vi "warmup.vi"(0 "VISA resource name":refnum<visa-resource-name>, 1 "SMU1 Terminal":string(combo)="Source", 5 "error in (no error)":errorcluster, 12 "Sweep 0":T1={"DorG_0"="", "Vvar_0_start"=0.0, "Vvar_0_step"=0.0, "Vvar_0_Stop"=0.0, "Vvar_1_start "=0.0, "Drain Current Compliance"=1e-06, "Gate Current Compliance 0"=1e-06, "Vvar_0_holdtime"=0.0, "Vvar-0_delaytime"=0.0, "IntPts_0"=100.0, "Set Swe_0_Mode"="", "Sweep Spacing_0"=""}) -> (14 "VISA resource name out":refnum<visa-resource-name>, 15 "Recorded_data":dbl[][](array[numeric]), 19 "error out":errorcluster)   [LabVIEW 2021]
panel:
  out "V Slave":string
  out "V Lead":string
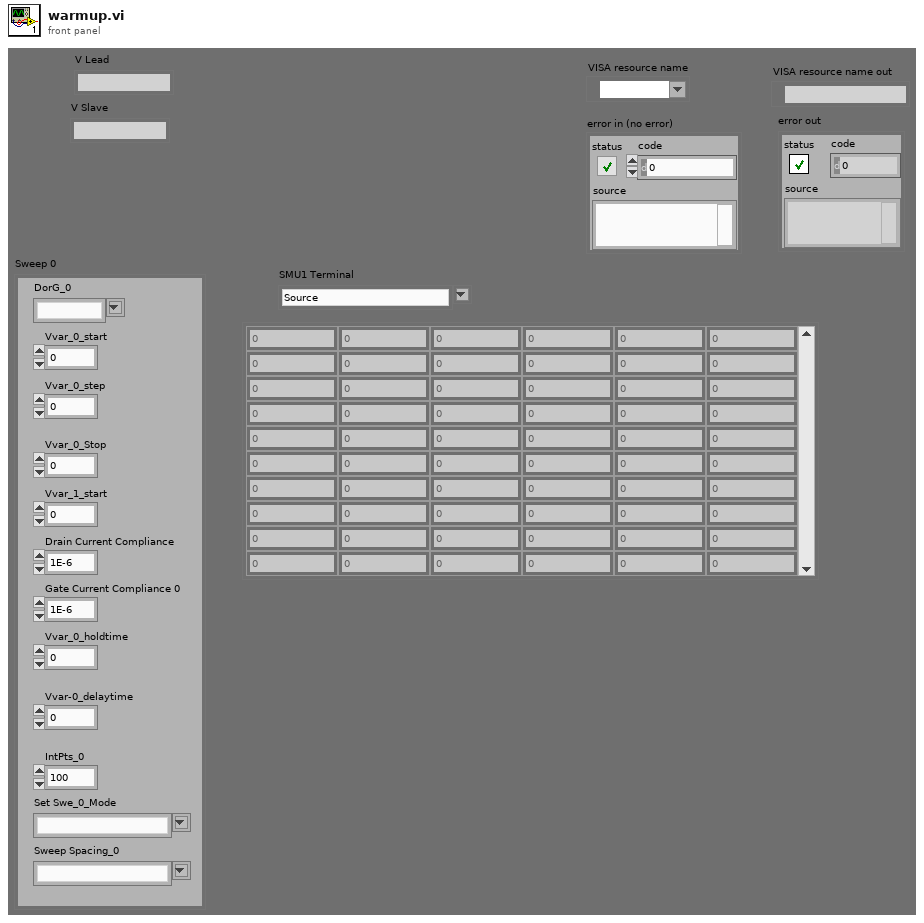
[diagram p1: front panel]
types:
  T1 = cluster{"DorG_0":string, "Vvar_0_start":dbl, "Vvar_0_step":dbl, "Vvar_0_Stop":dbl, "Vvar_1_start ":dbl, "Drain Current Compliance":dbl, "Gate Current Compliance 0":dbl, "Vvar_0_holdtime":dbl, "Vvar-0_delaytime":dbl, "IntPts_0":dbl, "Set Swe_0_Mode":string, "Sweep Spacing_0":string}
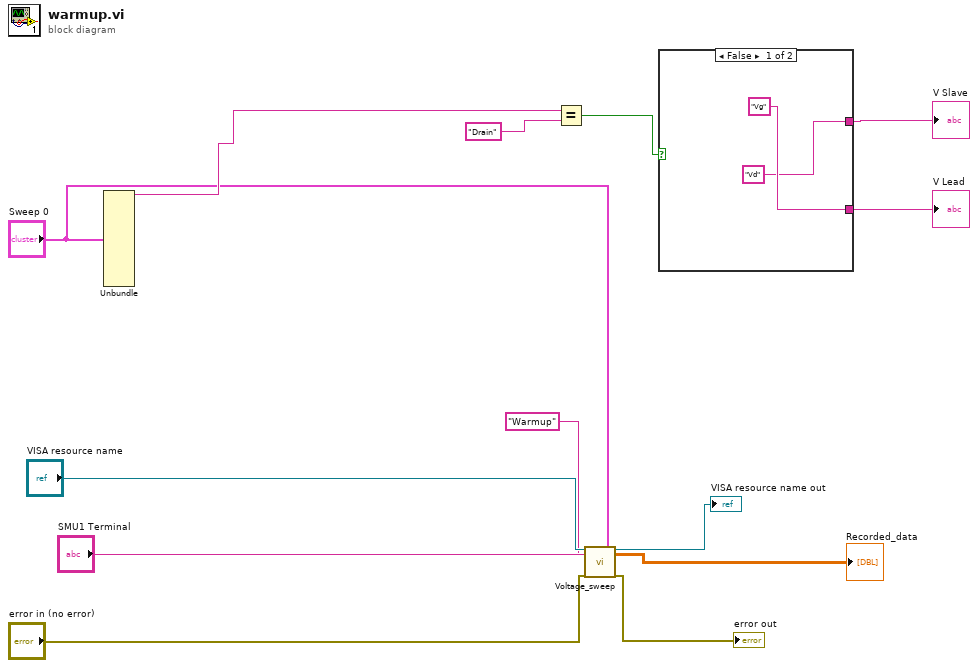
[diagram p0: block diagram]
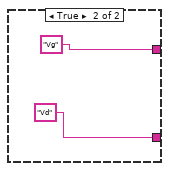
[diagram p2: hidden frame]
diagram:
  n1 = Unbundle("Sweep 0") -> ("DorG_0"=w9:string)  [unwired: 11 out]
  n2 = Equal?(x=w9, y="Drain") -> (x = y?=w13:bool)
  n3 = call "Voltage_sweep.vi"("VISA resource name"="VISA resource name", "smu_1_port"="SMU1 Terminal", "error in (no error)"="error in (no error)", "Queue_name_for_multiple_streams"="Warmup", "Sweep 0"="Sweep 0") -> ("VISA resource name out"=→"VISA resource name out":refnum<visa-resource-name>, "Recorded_data"=→"Recorded_data":dbl[][], "error out"=→"error out":errorcluster)  [unwired: 12 in]
  n4 = case shown="False" w13 {
    tunnel: ["Vd" "Vg"] -> w10
    tunnel: ["Vg" "Vd"] -> w11
    frame False {
    }
    frame True {
    }
  }
  "V Lead" <- w11
  "V Slave" <- w10
